vi "Example - Call endpoint asynchronously.vi"() -> ()   [LabVIEW 2020, in "wamplv.lvlib"]
uses:
  wamplv.lvlib
  WAMP Client/WAMP Client.lvclass/WAMP Client.ctl
  0748ca70-c771-45d1-a049-0e3afa802e33.vi
  WAMP Client/API/WAMP/JSON/Call (async) JSON.vi
  WAMP Client/Private/SubVIs/Raise Internal Message.vi
  WAMP Client/API/WAMP/JSON/Call (async) JSON.vi/44dd0fb6-e4b1-424e-8704-d5c62803e1d5.vi
  WAMP Client/API/Is Connected.vi
  <vilib>/JDP Science/JSONtext/Variant to JSON Text.vi
  <vilib>/Utility/error.llb/Error Cluster From Error Code.vi
  WAMP Client/Private/SubVIs/Check URI.vi
  <vilib>/JDP Science/JSONtext/LVClass Serializer/JSONtext LVClass Serializer.lvclass
  WAMP Client/WAMP Client.lvclass
panel:
  out "Result ArgumentKw Payload":string
  out "Result Arguments Payload":string
  in  "Call Arguments":string[](array[string])
  in  "Topic URI":string="test.topic"
  in  "Realm":string="default_realm"
  in  "Router URL":string="ws://localhost:8080/"
  # "Example: call endpoint asynchronously"
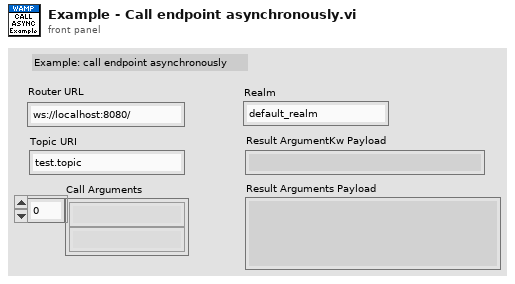
[diagram p1: front panel]
types:
  T1 = typedef "wamplv.lvlib/WAMP Client.lvclass/RESULT payload.ctl" = cluster{"Arguments Payload":string, "ArgumentKw Payload":string, "Topic":string, "Combined Error":T2}
  T2 = typedef "wamplv.lvlib/WAMP Client.lvclass/Combined error.ctl" = cluster{"Error?":bool, "WAMP Error":T3, "Error":errorcluster}
  T3 = typedef "wamplv.lvlib/WAMP Client.lvclass/WAMP error.ctl" = cluster{"Details":string, "ArgumentKw Payload":string, "Error?":bool, "Error URI":string, "Arguments Payload":string}
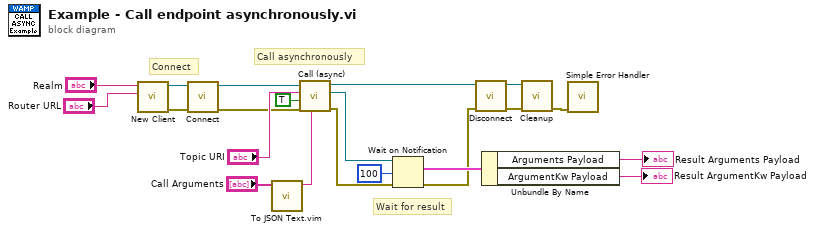
[diagram p0: block diagram]
diagram:
  # "Wait for result"
  # "Call asynchronously"
  # "Connect"
  n1 = call "New Client.vi"("Address"="Router URL", "Realm"="Realm") -> ("error out"=w16:errorcluster, "WAMP client out"=w19:refnum<class "WAMP Client.lvclass">)  [unwired: 8 in]
  n2 = call "Connect.vi"("error in"=w16, "WAMP Client in"=w19) -> ("error out"=w11:errorcluster, "WAMP Client out"=w13:refnum<class "WAMP Client.lvclass">)  [unwired: 8 in]
  n3 = call "To JSON Text.vim"("Anything"="Call Arguments") -> ("<JSON>"=w10:string)  [unwired: 9 in, 1 out]
  n4 = call-poly "Call (async).vi"("Arguments"=w10, "error in (no error)"=w11, "Notify result"=TRUE, "Topic URI"="Topic URI", "WAMP Client in"=w13) -> ("error out"=w9:errorcluster, "Call result notifier"=w8:refnum<notifier>, "WAMP Client out"=w2:refnum<class "WAMP Client.lvclass">)  [unwired: 4 in]
  n5 = Wait on Notification(notifier=w8, timeout in ms (-1)=100, error in (no error)=w9) -> (notification=w6:T1, error out=w3:errorcluster)  [unwired: 1 in, 2 out]
  n6 = call-dynamic "Disconnect.vi"("error in"=w3, "WAMP Client in"=w2) -> ("error out"=w15:errorcluster, "WAMP Client out"=w18:refnum<class "WAMP Client.lvclass">)  [unwired: 8 in]
  n7 = Unbundle By Name(w6) -> ("Arguments Payload"=→"Result Arguments Payload":string, "ArgumentKw Payload"=→"Result ArgumentKw Payload":string)
  n8 = call-dynamic "Cleanup.vi"("error in"=w15, "WAMP Client in"=w18) -> ("error out"=w17:errorcluster)  [unwired: 8 in, 1 out]
  n9 = call <vilib>:"Simple Error Handler.vi"("error in (no error)"=w17) -> ()  [unwired: 4 in, 5 out]
